vi "Inspect Folder.vi"(6 "Extensions (vi, vim, vit)":string[](array[string])=["vi", "vim", "vit"], 7 "Inspector Config":T2, 8 "error in (no error)":errorcluster, 11 "Folder":path) -> (0 "error out":errorcluster, 2 "Good":bool, 3 "Results":T1[](array[typedef]))   [LabVIEW 2020, in "SoL Inspector.lvlib"]
uses:
  SoL Inspector.lvlib
  Inspector Config.ctl
  Inspection.ctl
  Inspection Result.ctl
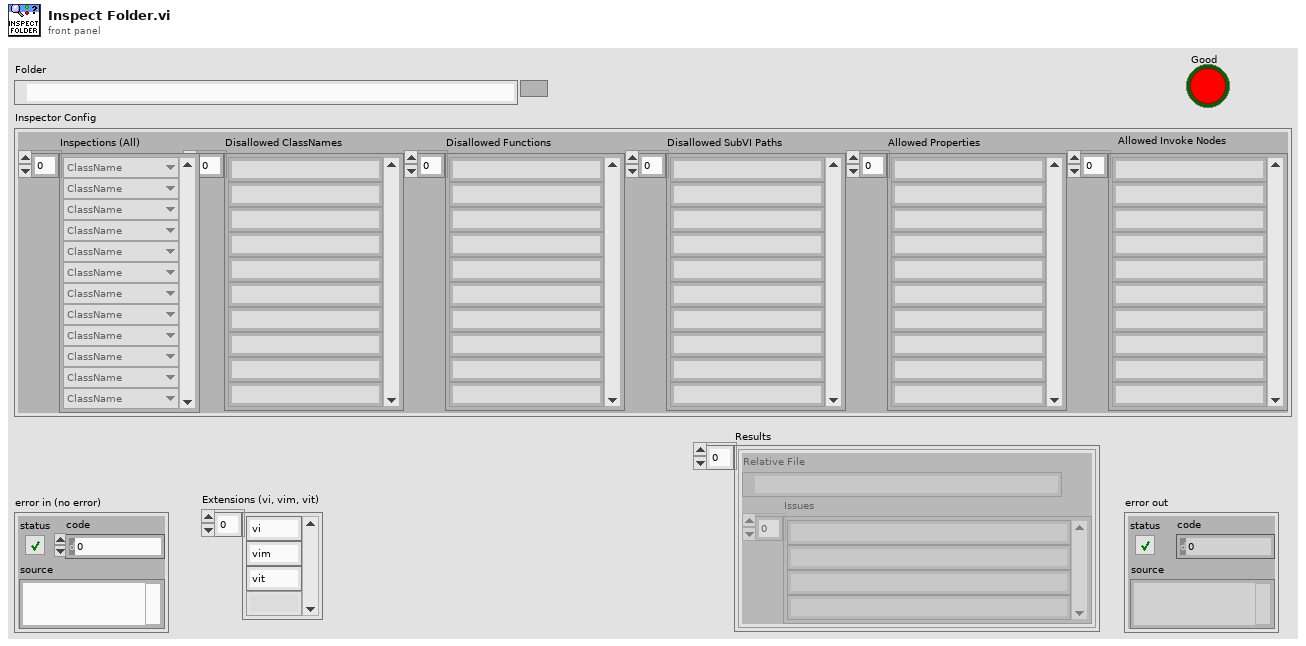
[diagram p1: front panel]
types:
  T1 = typedef "SoL Inspector.lvlib/Inspection Result.ctl" = cluster{"Relative File":path, "Issues":string[]}
  T2 = typedef "SoL Inspector.lvlib/Inspector Config.ctl" = cluster{"Inspections (All)":T3[], "Disallowed ClassNames":string[], "Disallowed Functions":string[], "Disallowed SubVI Paths":string[], "Allowed Properties":string[], "Allowed Invoke Nodes":string[]}
  T3 = typedef "SoL Inspector.lvlib/Inspection.ctl" = enum16{"ClassName", "Functions", "CallLibrary", "SubVIs", "FileIO", "Invoke Nodes", "Properties", "Growable Functions"}
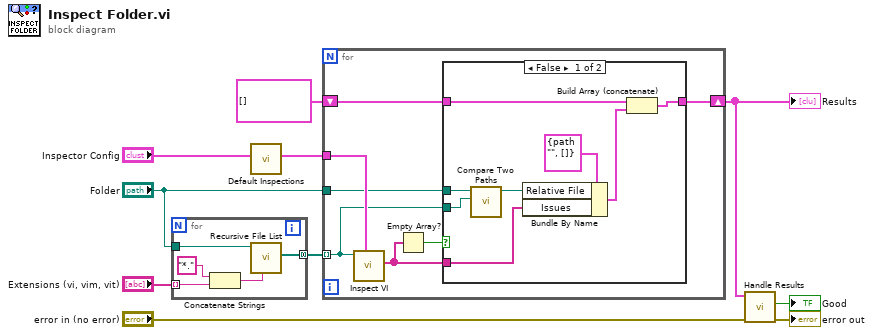
[diagram p0: block diagram]
diagram:
  n1 = for {
    tunnel: "Folder" -> [w15]
    tunnel: "Extensions (vi, vim, vit)" -> [w13] mode=indexing
    tunnel: [w11] -> w3 mode=concatenating
    n2 = Concatenate Strings("*.", w13) -> (w12:string)
    n3 = call <vilib>:"Recursive File List.vi"("pattern"=w12, "Folder Path"=w15) -> ("All Files in Dir"=w11:path[])  [unwired: 5 in, 4 out]
  }
  n4 = call "Default Inspections.vi"("Inspector Config in"="Inspector Config") -> ("Inspector Config"=w1:T2)  [unwired: 10 in]
  n5 = for {
    tunnel: w3 -> [w18] mode=indexing
    tunnel: w1 -> [w22]
    shift-right: [w17] -> w8
    shift-left: T1[] [] ("Array") -> [w20]
    tunnel: "Folder" -> [w19]
    n6 = call "Inspect VI.vi"("Inspector Config"=w22, "VI Path"=w18) -> ("Issues"=w16:string[])  [unwired: 7 in, 2 out]
    n7 = Empty Array?(array=w16) -> (empty?=w21:bool)
    n8 = case shown="False" w21 {
      tunnel: w20 -> [w25 w31]
      tunnel: w19 -> [w30 _]
      tunnel: w18 -> [w29 _]
      tunnel: [w23 w31] -> w17
      tunnel: w16 -> [w26 _]
      frame False {
        n9 = call <vilib>:"Compare Two Paths.vi"("Path 2"=w29, "Path 1"=w30) -> ("Relative Path from 1 to 2"=w27:path)  [unwired: 6 in, 3 out]
        n10 = Bundle By Name(cluster=T1 {"Relative File"=path "", "Issues"=[]} ("Inspection Result"), "Relative File"=w27, "Issues"=w26) -> (w24:T1)
        n11 = Build Array (concatenate)(w25, w24) -> (w23:T1[])
      }
      frame True {
      }
    }
  }
  "Results" <- w8
  n12 = call "Handle Results.vi"("error in (no error)"="error in (no error)", "Results"=w8) -> ("error out"=→"error out":errorcluster, "Result"=→"Good":bool)  [unwired: 8 in]
